vi "Available Connections.vi"() -> (3 "Available Types":T1[](array[typedef]))   [LabVIEW 2020, in "LV-Term.lvlib" / "LV-Term App.lvclass"]
uses:
  LV-Term App.lvclass
  Available Type.ctl
  <vilib>/IlluminatedG/lv-stream/Endpoint/Endpoint.lvclass
  <vilib>/IlluminatedG/IG Serial Stream/Stream-Serial/Serial Client/Serial Client.lvclass
  C:/Program Files (x86)/National Instruments/LabVIEW 2020/vi.lib/IlluminatedG/lv-stream/Endpoint/Endpoint.lvclass
  <vilib>/IlluminatedG/lv-stream-tcp/TCP Client/TCP Client.lvclass
  SerialConfigPanel/SerialConfigPanel.lvclass
  C:/Program Files (x86)/National Instruments/LabVIEW 2020/vi.lib/IlluminatedG/IG OOPanel/OOPanel/Panel/Panel.lvclass
  TCPConfigPanel/TCPConfigPanel.lvclass
  LV-Term App.lvclass/LV-Term App.ctl
  ConfigPanel/ConfigPanel.lvclass
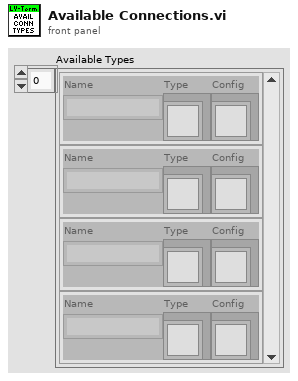
[diagram p1: front panel]
types:
  T1 = typedef "LV-Term.lvlib/LV-Term App.lvclass/Available Type.ctl" = cluster{"Name":string, "Type":refnum<class "Endpoint.lvclass">, "Config":refnum<class "ConfigPanel.lvclass">}
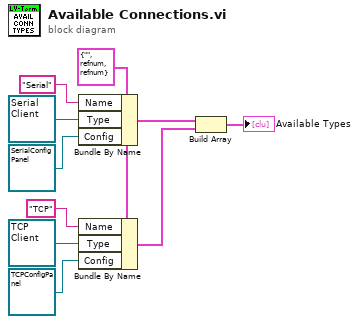
[diagram p0: block diagram]
diagram:
  w8 = T1 {"Name"="", "Type"=refnum, "Config"=refnum} ("Available Type")
  n1 = Bundle By Name(cluster=w8, "Name"="Serial", "Type"=refnum<class "Serial Client.lvclass"> refnum ("Stream-Serial.lvlib:Serial Client.lvclass"), "Config"=refnum<class "SerialConfigPanel.lvclass"> refnum ("LV-Term.lvlib:SerialConfigPanel.lvclass")) -> (w7:T1)
  n2 = Bundle By Name(cluster=w8, "Name"="TCP", "Type"=refnum<class "TCP Client.lvclass"> refnum ("TCP Client in"), "Config"=refnum<class "TCPConfigPanel.lvclass"> refnum ("LV-Term.lvlib:TCPConfigPanel.lvclass")) -> (w6:T1)
  n3 = Build Array(w7, w6) -> (→"Available Types":T1[])
